vi "rad_Get Target Info (Subnet) Wrapper.vi"(5 "Password":string, 6 "reduce discovery timeout (T)":bool=TRUE, 8 "error in (no error)":errorcluster, 10 "only installable systems (T)":bool=TRUE) -> (0 "error out":errorcluster, 3 "target information":T1[](array[typedef]) {"Primary NIC"."IP Address Request Mode" items=["Static"=1, "DHCP/Link-Local"=2, "Link-Local Only"=4, "DHCP Only"=8]})   [LabVIEW 2020]
uses:
  <vilib>/nisyscfg/nisyscfg.lvlib
  TypeDefs/rad_Target Information.ctl
  <vilib>/nisyscfg/Close (System).vi
  TypeDefs/rad_Target Network Settings.ctl
  <vilib>/nisyscfg/Find Systems.vi
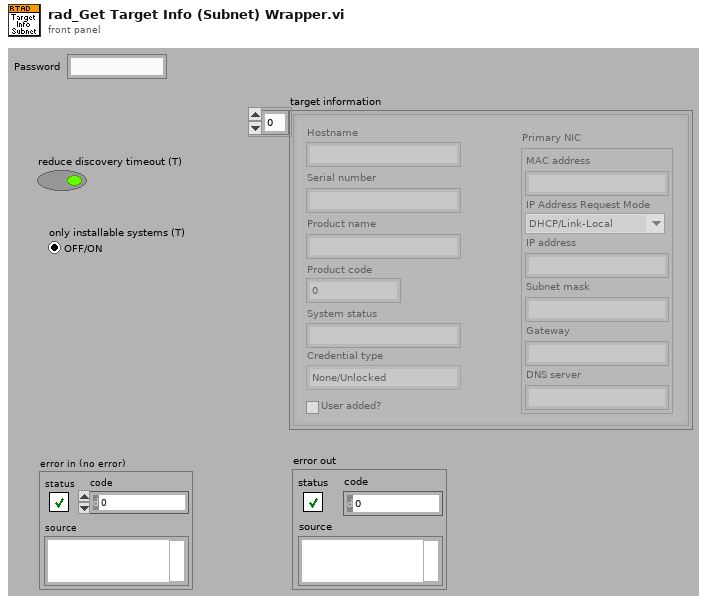
[diagram p1: front panel]
types:
  T1 = typedef "rad_Target Information.ctl" = cluster{"Hostname":string, "Serial number":string, "Product name":string, "Product code":i32, "System status":string, "Credential type":enum16{"None/Unlocked", "FTP Password", "NIAuth Credentials"}, "User added?":bool, "Primary NIC":T2}
  T2 = typedef "rad_Target Network Settings.ctl" = cluster{"MAC address":string, "IP Address Request Mode":i32, "IP address":string, "Subnet mask":string, "Gateway":string, "DNS server":string}
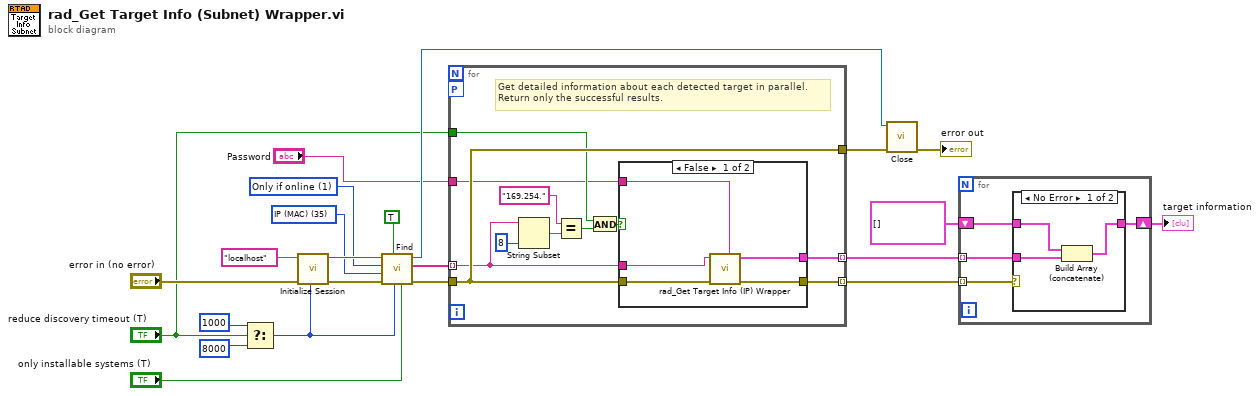
[diagram p0: block diagram]
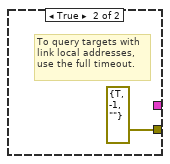
[diagram p3: hidden frame]
diagram:
  w18 = u32 35 items=["Hostname"=16, "Hostname (IP)"=18, "Hostname (MAC)"=19, "IP"=32, "IP (Hostname)"=33, "IP (MAC)"=35, "MAC"=48, "MAC (Hostname)"=49, "MAC (IP)"=50] ("output (hostname and IP)")
  w19 = u32 1 items=["None"=0, "Only if online"=1, "All"=3] ("include cached results (all)")
  n1 = Select(t=u32 1000, s="reduce discovery timeout (T)", f=u32 8000) -> (s? t:f=w2:u32)
  n2 = call <vilib>:"Initialize Session.vi"("Connect Timeout (4000 ms)"=w2, "error in (no error)"="error in (no error)", "Target (localhost)"="localhost") -> ("error out"=w17:errorcluster, "Session out"=w21:refnum<k21>)  [unwired: 7 in]
  n3 = call-poly <vilib>:"Find.vi"("Only Installable Systems (F)"="only installable systems (T)", "Timeout (4000 ms)"=w2, "Detect Online Systems (T)"=TRUE ("detect online systems (T)"), "error in (no error)"=w17, "Output (Hostname and IP)"=w18, "Include Cached Results (all)"=w19, "Session in (localhost)"=w21) -> ("error out"=w14:errorcluster, "Detected Systems"=w16:string[], "Session out"=w12:refnum<k21>)  [unwired: 2 in]
  n4 = for {
    tunnel: w16 -> [w30] mode=indexing
    tunnel: w14 -> [w33]
    tunnel: [w33] -> w13
    workers-P: _ -> [_]
    tunnel: [w32] -> w9 mode=indexing
    tunnel: [w31] -> w10 mode=indexing
    tunnel: "reduce discovery timeout (T)" -> [w24]
    tunnel: "Password" -> [w23]
    # "Get detailed information about each detected target in parallel.\nReturn only the successful results."
    n5 = String Subset(string=w30, length (rest)=8 ("length (rest)")) -> (substring=w27:string)  [unwired: 1 in]
    n6 = Equal?(x="169.254.", y=w27) -> (x = y?=w25:bool)
    n7 = And(x=w24, y=w25) -> (x .and. y?=w26:bool)
    n8 = case shown="False" w26 {
      tunnel: w33 -> [w38 _]
      tunnel: [w37 errorcluster {"status"=TRUE, "code"=-1, "source"=""} ("error out")] -> w32
      tunnel: [w36 _] -> w31
      tunnel: w30 -> [w35 _]
      tunnel: w23 -> [w34 _]
      frame False {
        n9 = call "rad_Get Target Info (IP) Wrapper.vi"("Password"=w34, "error in (no error)"=w38, "target address"=w35) -> ("error out"=w37:errorcluster, "Target settings"=w36:T1)  [unwired: 7 in]
      }
      frame True {
        # "To query targets with\nlink local addresses,\nuse the full timeout."
      }
    }
  }
  n10 = call-poly <vilib>:"Close.vi"("error in (no error)"=w13, "Session in"=w12) -> ("error out"=→"error out":errorcluster)  [unwired: 9 in]
  n11 = for {
    tunnel: w10 -> [w41] mode=indexing
    tunnel: w9 -> [w43] mode=indexing
    shift-right: [w40] -> w7
    shift-left: T1[] [] -> [w42]
    n12 = case shown="No Error" w43 {
      tunnel: w42 -> [w46 w47]
      tunnel: w41 -> [w45 _]
      tunnel: [w44 w47] -> w40
      frame No Error {
        n13 = Build Array (concatenate)(w46, w45) -> (w44:T1[])
      }
      frame Error {
      }
    }
  }
  "target information" <- w7
